vi "XYgraph_Create.vi"(0 "reference in":refnum<class "XYgraph.lvclass">, 2 "FPref":T1, 5 "error in (no error)":errorcluster) -> (14 "reference out":refnum<class "XYgraph.lvclass">, 19 "error out":errorcluster)   [LabVIEW 2019, in "XYgraph.lvclass"]
doc: "Constructor."
uses:
  XYgraph.lvclass
  C:/Program Files (x86)/National Instruments/LabVIEW 2019/vi.lib/addons/_AddQ/G#Object/G#Object.lvclass
  XY graph ref.ctl
  <vilib>/addons/_AddQ/G#Object/G#Object.lvclass
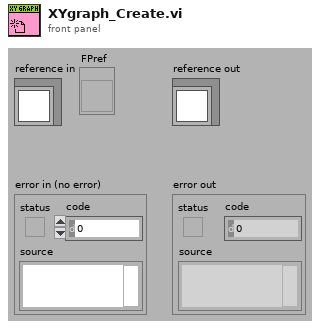
[diagram p1: front panel]
types:
  T1 = typedef "XYgraph.lvclass/XY graph ref.ctl" = refnum<vi>
  T2 = typedef "XYgraph.lvclass/ObjectAttributesRef.ctl" = refnum<data-value>
  T3 = typedef "XYgraph.lvclass/ObjectAttributes.ctl" = cluster{"FPref":T1, "MyAttribute":dbl, "X multiplier":dbl, "Y multiplier":dbl, "X Scale name":string, "Y Scale name":string, "Fcurve metadata":T4, "Fcurve":refnum<class "Fcurve.lvclass">}
  T4 = typedef "Fcurve.lvclass/Metadata.ctl" = cluster{"dt (us)":dbl, "Dec Factor":dbl, "Z piezo Sensitivity (nm/V)":dbl, "K (N/m)":dbl, "Sp (V)":dbl, "Contact (ms)":dbl, "Zpos contact":dbl, "Vel_app (nm/s)":dbl, "Vel_ret (nm/s)":dbl, "deltaV (nm)":dbl, "Def_V0 (v)":dbl, "Piezo gain":dbl, "invOLS (nm/V)":dbl}
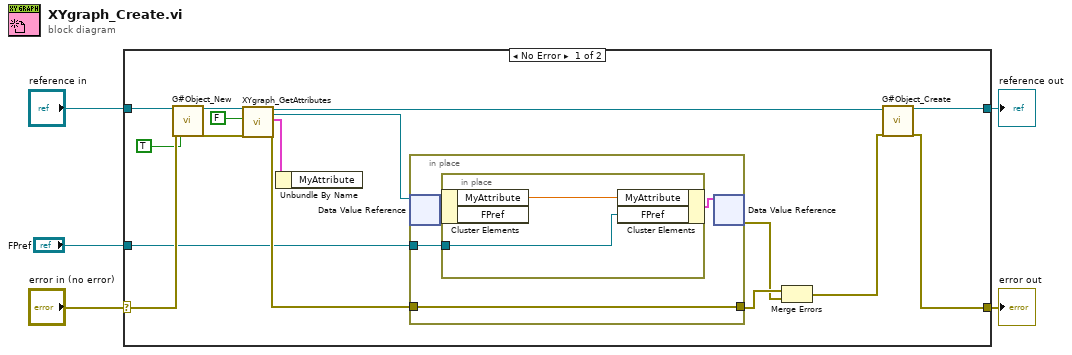
[diagram p0: block diagram]
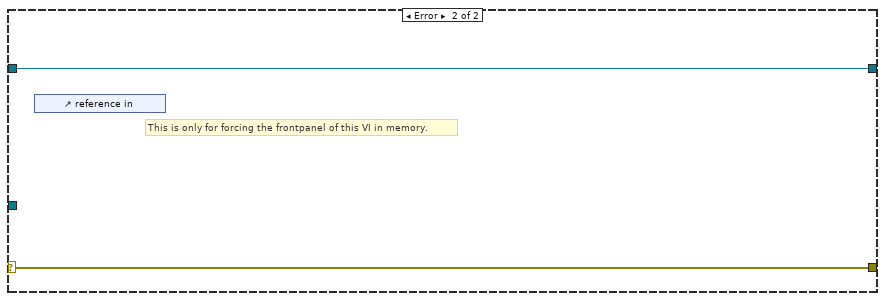
[diagram p2: hidden frame]
diagram:
  n1 = case shown="No Error" "error in (no error)" {
    selector: "error in (no error)" -> [w20 w29]
    tunnel: [w7 w29] -> w4
    tunnel: [w9 w28] -> w2
    tunnel: "reference in" -> [w21 w28]
    tunnel: "FPref" -> [w6 _]
    frame No Error {
      n2 = call <vilib>:"G#Object_New.vi"("reference in"=w21, "error in (no error)"=w20, "user counter (T)?"=TRUE ("User Counter")) -> ("reference out"=w13:refnum<class "XYgraph.lvclass">, "error out"=w12:errorcluster)  [unwired: 14 in, 1 out]
      n3 = call "XYgraph_GetAttributes.vi"("reference in"=w13, "return data? (T)"=FALSE ("return data"), "error in (no error)"=w12) -> ("reference out"=w10:refnum<class "XYgraph.lvclass">, "attributes ref"=w15:T2, "attributes"=w11:T3, "error out"=w16:errorcluster)  [unwired: 13 in]
      n4 = Unbundle By Name(w11) -> ()  [unwired: 1 out]
      n5 = in-place {
        in-place-border: w16 -> [w23]
        in-place-border: [w23] -> w18
        in-place-border: w6 -> [w22]
        n6 = in-place-dvr #1(w15) -> (w24:T3)  [unwired: 1 out]
        n7 = in-place {
          in-place-border: w22 -> [w26]
          n8 = in-place-cluster #2(w24) -> ("MyAttribute"=w27:dbl)  [unwired: 1 out]
          n9 = in-place-cluster #2("MyAttribute"=w27, "FPref"=w26) -> (w25:T3)
        }
        n10 = in-place-dvr #1(w25) -> (w17:errorcluster)  [unwired: 1 out]
      }
      n11 = Merge Errors(w18, w17) -> (w8:errorcluster)
      n12 = call-dynamic "G#Object_Create.vi"("reference in"=w10, "error in (no error)"=w8) -> ("reference out"=w9:refnum<class "XYgraph.lvclass">, "error out"=w7:errorcluster)  [unwired: 16 in]
    }
    frame Error {
      # "This is only for forcing the frontpanel of this VI in memory."
      n13 = control-ref of="reference in"() -> ()  [unwired: 1 out]
    }
  }
  "error out" <- w4
  "reference out" <- w2
